vi "Update Override Command.vi"(8 "error in":errorcluster, 10 "Plugin Overrides":T1, 11 "CoreOOB_Tx in":refnum<class "CIFCoreOOB_Tx.lvclass">) -> (0 "error out":errorcluster, 3 "CoreOOB_Tx out":refnum<class "CIFCoreOOB_Tx.lvclass">)   [LabVIEW 2021, in "CIFCoreOOB_Tx.lvclass"]
uses:
  CIFCoreOOB_Tx.lvclass
  D:/dev/CIF-LVCore/src/CIFUtilities/CIFOutOfBand/CIFOutOfBand.lvclass
  Common/Typedef/Plugin Overrides.ctl
  Common/Typedef/Timing Overrides.ctl
  CIFUtilities/CIFOutOfBand/CIFOutOfBand.lvclass/CIFOutOfBand.ctl
  Typedef/Template Payload.ctl
  Common/Typedef/Plugin Status.ctl
  Common/Typedef/Plugin State.ctl
  Common/Typedef/Timing Statistics.ctl
  Common/Typedef/Timing Stats Base.ctl
  Common/Typedef/FIFO Statistics.ctl
  Common/Typedef/Simple Error.ctl
  Common/Typedef/Monitor Doubles.ctl
  Common/Typedef/Monitor U64.ctl
  Common/Typedef/Monitor I64.ctl
  Typedef/OOB Core Commands.ctl
  CIFCoreOOB_Tx.lvclass/CIFCoreOOB_Tx.ctl
  CIFUtilities/CIFOutOfBand/CIFOutOfBand.lvclass
  Common/CIFCoreCommon.lvlib
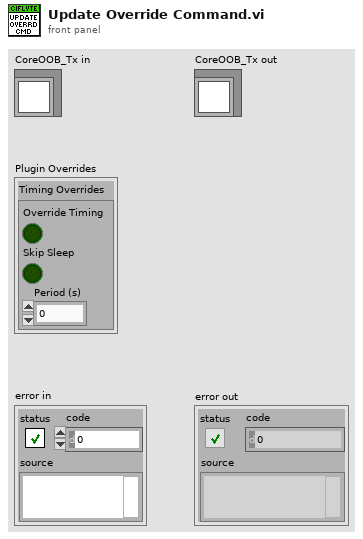
[diagram p1: front panel]
types:
  T1 = typedef "CIFCoreCommon.lvlib/Plugin Overrides.ctl" = cluster{"Timing Overrides":T2}
  T2 = typedef "CIFCoreCommon.lvlib/Timing Overrides.ctl" = cluster{"Override Timing":bool, "Skip Sleep":bool, "Period (s)":dbl}
  T3 = typedef "CIFCoreOOB_Tx.lvclass/Template Payload.ctl" = cluster{"Status":T4, "Plugin Overrides":T1}
  T4 = typedef "CIFCoreCommon.lvlib/Plugin Status.ctl" = cluster{"State":T5, "Timing Statistics (us)":T6, "FIFO Statistics (us)":T8, "error":T9, "Monitor Doubles":T10, "Monitor U64":T11, "Monitor I64":T12, "Cleanup":T7, "Create":i32, "Destroy":i32}
  T5 = typedef "CIFCoreCommon.lvlib/Plugin State.ctl" = enum32{"Null", "Creating", "Listening", "Running", "CleaningUp", "Destroying"}
  T6 = typedef "CIFCoreCommon.lvlib/Timing Statistics.ctl" = cluster{"Period":T7, "Wake Error":T7, "Execute":T7, "Housekeep":T7, "Idle":T7}
  T7 = typedef "CIFCoreCommon.lvlib/Timing Stats Base.ctl" = cluster{"Max":i32, "Min":i32}
  T8 = typedef "CIFCoreCommon.lvlib/FIFO Statistics.ctl" = cluster{"From T0":T7, "From Previous Plugin":T7, "Output Error":T7}
  T9 = typedef "CIFCoreCommon.lvlib/Simple Error.ctl" = cluster{"status":bool, "code":i32}
  T10 = typedef "CIFCoreCommon.lvlib/Monitor Doubles.ctl" = cluster{"1":dbl, "2":dbl, "3":dbl, "4":dbl}
  T11 = typedef "CIFCoreCommon.lvlib/Monitor U64.ctl" = cluster{"1":u64, "2":u64, "3":u64, "4":u64}
  T12 = typedef "CIFCoreCommon.lvlib/Monitor I64.ctl" = cluster{"1":i64, "2":i64, "3":i64, "4":i64}
  T13 = typedef "CIFCoreOOB_Tx.lvclass/OOB Core Commands.ctl" = enum8{"Status", "Overrides"}
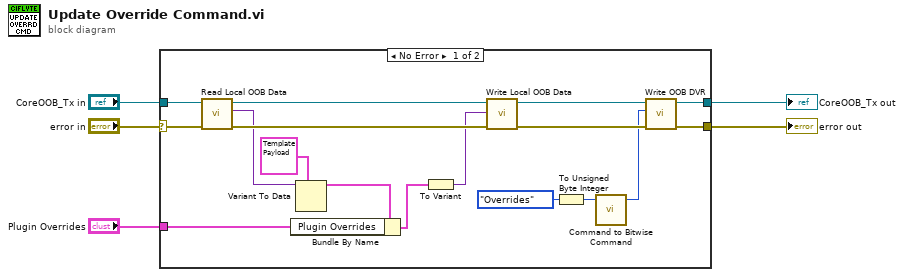
[diagram p0: block diagram]
diagram:
  n1 = case shown="No Error" "error in" {
    selector: "error in" -> [w20 w24]
    tunnel: [w21 w24] -> w4
    tunnel: "CoreOOB_Tx in" -> [w19 w23]
    tunnel: [w22 w23] -> w2
    tunnel: "Plugin Overrides" -> [w6 _]
    frame No Error {
      n2 = call "Read Local OOB Data.vi"("error in"=w20, "OOB in"=w19) -> ("error out"=w10:errorcluster, "Local OOB Data"=w8:variant, "OOB out"=w11:refnum<class "CIFCoreOOB_Tx.lvclass">)  [unwired: 7 in]
      n3 = Variant To Data(type=T3 {"Status"={"State"=enum."Null", "Timing Statistics (us)"={"Period"={"Max"=0, "Min"=1000}, "Wake Error"={"Max"=3, "Min"=2}, "Execute"={"Max"=994, "Min"=992}, "Housekeep"={"Max"=2, "Min"=2}, "Idle"={"Max"=0, "Min"=0}}, "FIFO Statistics (us)"={"From T0"={"Max"=0, "Min"=0}, "From Previous Plugin"={"Max"=0, "Min"=0}, "Output Error"={"Max"=0, "Min"=0}}, "error"={"status"=FALSE, "code"=0}, "Monitor Doubles"={"1"=0.0, "2"=0.0, "3"=0.0, "4"=0.0}, "Monitor U64"={"1"=0, "2"=0, "3"=0, "4"=0}, "Monitor I64"={"1"=0, "2"=0, "3"=0, "4"=0}, "Cleanup"={"Max"=0, "Min"=0}, "Create"=0, "Destroy"=0}, "Plugin Overrides"={"Timing Overrides"={"Override Timing"=FALSE, "Skip Sleep"=FALSE, "Period (s)"=0.0}}} ("Template Payload"), Variant=w8) -> (data=w13:T3)  [unwired: 1 in, 1 out]
      n4 = Bundle By Name(cluster=w13, "Plugin Overrides"=w6) -> (w12:T3)
      n5 = To Variant(anything=w12) -> (Variant=w9:variant)
      n6 = call "Write Local OOB Data.vi"("error in"=w10, "Local OOB Data"=w9, "OOB in"=w11) -> ("error out"=w18:errorcluster, "OOB out"=w17:refnum<class "CIFCoreOOB_Tx.lvclass">)  [unwired: 7 in]
      n7 = To Unsigned Byte Integer(number=OOB_Core_Commands."Overrides" ("OOB Main Commands")) -> (unsigned 8bit integer=w16:u8)
      n8 = call "Command to Bitwise Command.vi"("OOB Command"=w16) -> ("bit command"=w15:u64)  [unwired: 3 in]
      n9 = call "Write OOB DVR.vi"("error in"=w18, "Commands (bitwise)"=w15, "OOB in"=w17) -> ("error out"=w21:errorcluster, "OOB out"=w22:refnum<class "CIFCoreOOB_Tx.lvclass">)  [unwired: 7 in]
    }
    frame Error {
    }
  }
  "error out" <- w4
  "CoreOOB_Tx out" <- w2
